vi "Calculate A-Weighted Noise.vi"(0 "Waveform in":waveform(dbl)[](array[waveform]), 5 "fmin (Hz)":dbl, 7 "fmax (Hz)":dbl, 9 "Window(Rectangle)":T1 items=["Rectangle"=0, "Hanning"=1, "Hamming"=2, "Blackman-Harris"=3, "Exact Blackman"=4, "Blackman"=5, "Flat Top"=6, "4 Term B-Harris "=7, "7 Term B-Harris"=8, "Low Sidelobe"=9, "Blackman Nuttall"=11, "Triangle"=30, "Bartlett-Hanning"=31, "Bohman"=32, "Parzen"=33, "Welch"=34, "Kaiser"=60, "Dolph-Chebyshev"=61, "Gaussian"=62], 11 "error in":errorcluster) -> (4 "Noise (dB A-weighted)":dbl[](array[numeric]), 15 "error out":errorcluster)   [LabVIEW 2020]
doc: "This VI helps to calculate the A-weighted Noise in the waveform"
uses:
  <vilib>/Analysis/4window.llb/windowTd.ctl
  <vilib>/measure/maspectr.llb/FFT Power Spectrum and PSD for 1 Chan.vi
  <vilib>/measure/NI_MAPro.lvlib
  <vilib>/Analysis/NI_AALPro.lvlib
panel:
  out "A-Weighted Power spectrum":cluster{"f0":dbl, "df":dbl, "magnitude":dbl[]}[](graph)
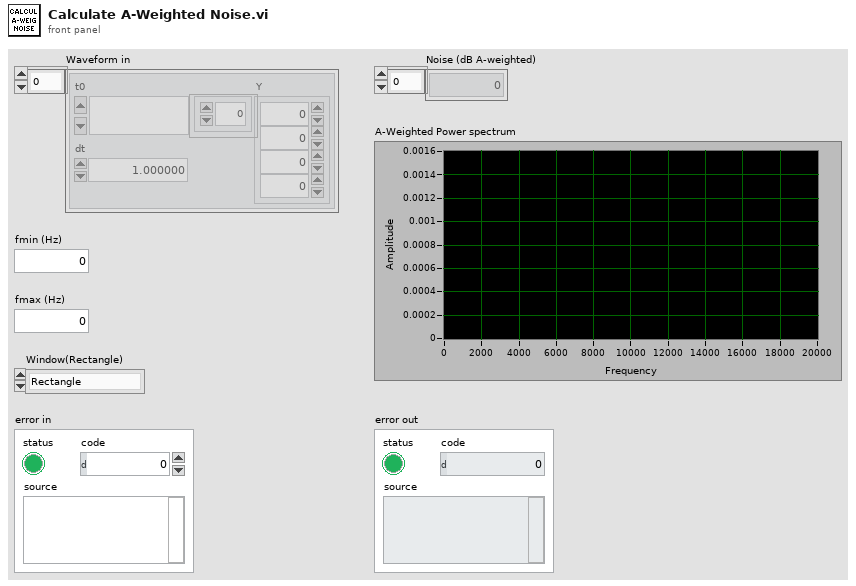
[diagram p1: front panel]
types:
  T1 = typedef "NI_AALPro.lvlib/windowTd.ctl" = u32
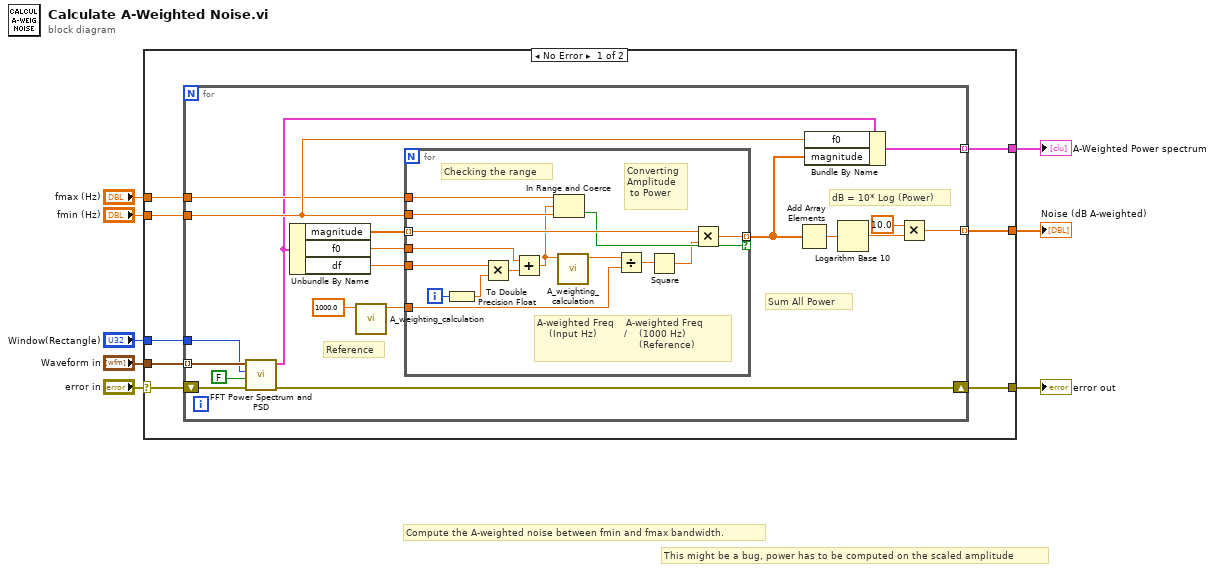
[diagram p0: block diagram]
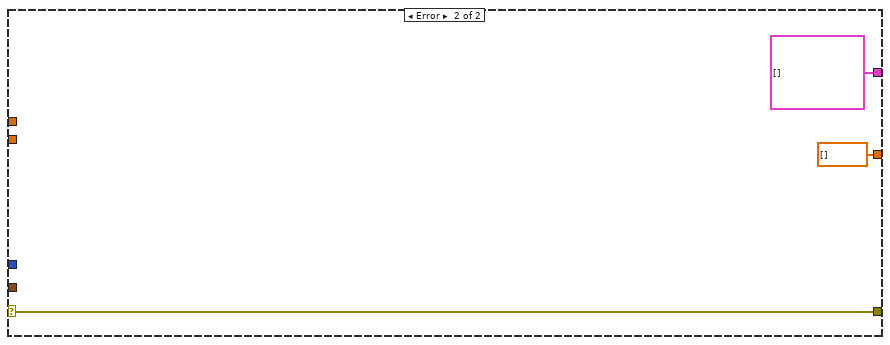
[diagram p2: hidden frame]
diagram:
  # "This might be a bug, power has to be computed on the scaled amplitude"
  # "Compute the A-weighted noise between fmin and fmax bandwidth."
  n1 = case shown="No Error" "error in" {
    selector: "error in" -> [w9 w53]
    tunnel: [w16 dbl[] []] -> w8
    tunnel: "fmin (Hz)" -> [w15 _]
    tunnel: "fmax (Hz)" -> [w14 _]
    tunnel: [w13 cluster{"f0":dbl, "df":dbl, "magnitude":dbl[]}[] []] -> w5
    tunnel: "Waveform in" -> [w12 _]
    tunnel: "Window(Rectangle)" -> [w11 _]
    tunnel: [w10 w53] -> w2
    frame No Error {
      n2 = for {
        tunnel: [w35] -> w16 mode=indexing
        tunnel: w15 -> [w34]
        tunnel: w14 -> [w33]
        tunnel: [w32] -> w13 mode=indexing
        tunnel: w12 -> [w31] mode=indexing
        tunnel: w11 -> [w30]
        shift-right: [w18] -> w10
        shift-left: w9 -> [w17]
        # "Sum All Power"
        # "Reference"
        # "dB = 10* Log (Power)"
        n3 = call-poly <vilib>:"FFT Power Spectrum and PSD.vi"("error in (no error)"=w17, "dB On (F)"=FALSE, "window"=w30, "time signal"=w31) -> ("error out"=w18:errorcluster, "Power Spectrum / PSD"=w21:cluster{"f0":dbl, "df":dbl, "magnitude":dbl[]})  [unwired: 4 in, 2 out]
        n4 = Unbundle By Name(w21) -> ("magnitude"=w28:dbl[], "f0"=w29:dbl, "df"=w22:dbl)
        n5 = call "A_weighting_calculation.vi"("Frequency"=1000.0) -> ("Ra(f)"=w19:dbl)  [unwired: 9 in, 1 out]
        n6 = for {
          tunnel: w34 -> [w50]
          tunnel: w29 -> [w41]
          tunnel: w28 -> [w48] mode=indexing
          tunnel: w33 -> [w49]
          tunnel: [w47] -> w24 mode=indexing if=w46
          tunnel: w22 -> [w40]
          tunnel: w19 -> [w38]
          i -> [w45]
          # "Converting\nAmplitude\n to Power"
          # "Checking the range"
          # "A-weighted Freq    A-weighted Freq \n    (Input Hz)         /    (1000 Hz)\n                                  (Reference)"
          n7 = To Double Precision Float(number=w45) -> (double precision float=w44:dbl)
          n8 = Multiply(x=w40, y=w44) -> (x*y=w43:dbl)
          n9 = Add(x=w41, y=w43) -> (x+y=w42:dbl)
          n10 = In Range and Coerce(upper limit=w49, x=w42, lower limit=w50) -> (In Range?=w46:bool)  [unwired: 1 out]
          n11 = call "A_weighting_calculation.vi"("Frequency"=w42) -> ("Ra(f)"=w39:dbl)  [unwired: 9 in, 1 out]
          n12 = Divide(x=w39, y=w38) -> (x/y=w37:dbl)
          n13 = Square(x=w37) -> (x^2=w36:dbl)
          n14 = Multiply(x=w48, y=w36) -> (x*y=w47:dbl)
        }
        n15 = Add Array Elements(numeric array=w24) -> (sum=w23:dbl)
        n16 = Bundle By Name(cluster=w21, "f0"=w34, "magnitude"=w24) -> (w32:cluster{"f0":dbl, "df":dbl, "magnitude":dbl[]})
        n17 = Logarithm Base 10(1:w23) -> (0:w27:dbl)
        n18 = Multiply(x=10.0, y=w27) -> (x*y=w35:dbl)
      }
    }
    frame Error {
    }
  }
  "Noise (dB A-weighted)" <- w8
  "A-Weighted Power spectrum" <- w5
  "error out" <- w2
